vi "Unpack Write Request.vi"(11 "WriteRequest in":refnum<class "WriteRequest.lvclass">) -> (2 "Execution Handler":refnum<class "IWriteExecutionCallback.lvclass">, 3 "Packet":refnum<class "IPacket.lvclass">)   [LabVIEW 2019, in "MessagingInterfaces.lvlib" / "WriteRequest.lvclass"]
uses:
  <vilib>/gpm_packages/@cs/Network-interface/Source/MessagingInterfaces/WriteRequest/WriteRequest.lvclass
  <vilib>/gpm_packages/@cs/Network-interface/Source/MessagingInterfaces/IPacket/IPacket.lvclass
  <vilib>/gpm_packages/@cs/Network-interface/Source/MessagingInterfaces/IWriteExecutionCallback/IWriteExecutionCallback.lvclass
  <vilib>/gpm_packages/@cs/Network-interface/Source/MessagingInterfaces/WriteRequest/WriteRequest.lvclass/WriteRequest.ctl
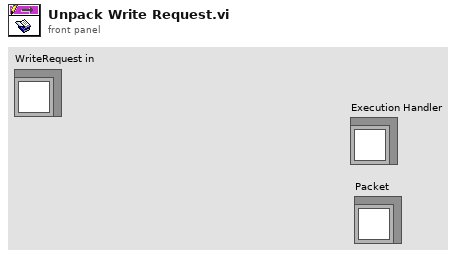
[diagram p1: front panel]
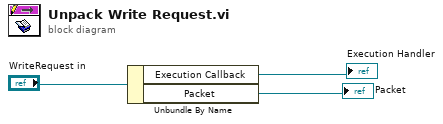
[diagram p0: block diagram]
diagram:
  n1 = Unbundle By Name("WriteRequest in") -> ("Execution Callback"=→"Execution Handler":refnum<class "IWriteExecutionCallback.lvclass">, "Packet"=→"Packet":refnum<class "IPacket.lvclass">)
